vi "Deinitialize Rigol.vi"(9 "VISA resource name":refnum<visa-resource-name>) -> (0 "error out":errorcluster)   [LabVIEW 2023, in "Rigol.lvlib"]
uses:
  Rigol.lvlib
  <instrlib>/RIGOL DP800 Series/RIGOL DP800 Series.lvlib
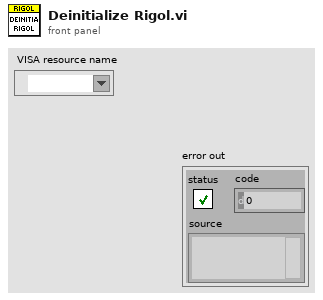
[diagram p1: front panel]
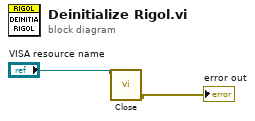
[diagram p0: block diagram]
diagram:
  n1 = call <instrlib>:"Close.vi"("VISA resource name"="VISA resource name") -> ("error out"=→"error out":errorcluster)  [unwired: 10 in]
